vi "GenerateWithoutData.vi"(8 "error in (no error)":errorcluster, 11 "String in":refnum<class "String.lvclass">) -> (0 "error out":errorcluster, 3 "String out":refnum<class "String.lvclass">)   [LabVIEW 2023, in "String.lvclass"]
uses:
  String.lvclass
  C:/Users/santharu.subramanian/Desktop/LOA New/Documents/LV New Assignments/Sender-Receiver/Classes/Data/Data.lvclass
  String.lvclass/String.ctl
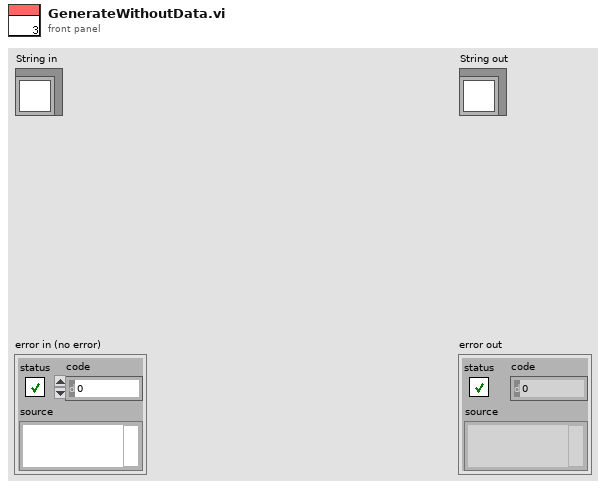
[diagram p1: front panel]
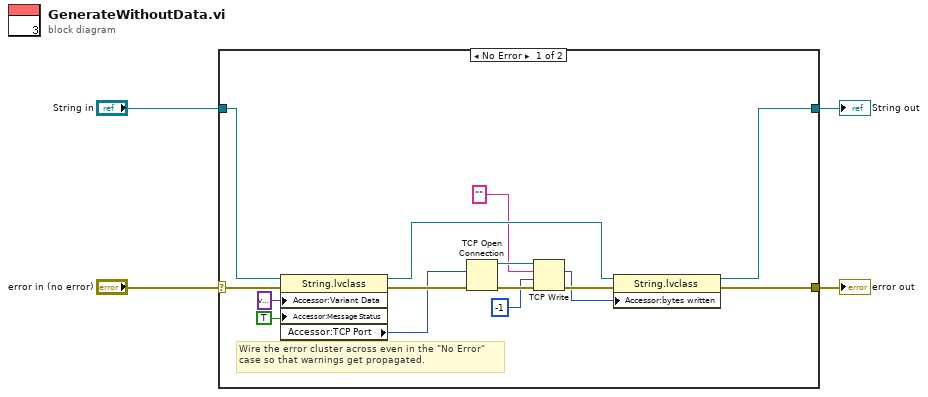
[diagram p0: block diagram]
diagram:
  n1 = case shown="No Error" "error in (no error)" {
    selector: "error in (no error)" -> [w19 w21]
    tunnel: [w8 w21] -> w3
    tunnel: [w7 w20] -> w1
    tunnel: "String in" -> [w18 w20]
    frame No Error {
      # "Wire the error cluster across even in the \"No Error\"\ncase so that warnings get propagated."
      n2 = property class="String.lvclass"(reference=w18, error in=w19, "Accessor:Variant Data"=variant ("Variant Data"), "Accessor:Message Status"=TRUE ("Message Status")) -> (reference out=w10:refnum<class "String.lvclass">, error out=w9:errorcluster, "Accessor:TCP Port"=w6:u16)
      n3 = TCP Open Connection(remote port or service name=w6, error in (no error)=w9) -> (connection ID=w14:refnum<k5>, error out=w15:errorcluster)  [unwired: 3 in]
      n4 = TCP Write(connection ID=w14, data in="", error in (no error)=w15, 9:-1 ("timeout ms (25000)")) -> (bytes written=w12:i32, error out=w13:errorcluster)  [unwired: 1 out]
      n5 = property class="String.lvclass"(reference=w10, error in=w13, "Accessor:bytes written"=w12) -> (reference out=w7:refnum<class "String.lvclass">, error out=w8:errorcluster)
    }
    frame Error {
    }
  }
  "error out" <- w3
  "String out" <- w1
